vi "Get Core Configuration.vi"(8 "error in":errorcluster, 11 "custom device":T1 format="%.0x") -> (0 "error out":errorcluster, 2 "configuration string":string, 3 "custom device out":T1 format="%.0x")   [LabVIEW 2020, in "Ballard ARINC 429 Hardware Configuration.lvlib"]
uses:
  Ballard ARINC 429 Hardware Configuration.lvlib
  <vilib>/NI VeriStand/Custom Device API/Custom Device Item Ref.ctl
  Constants.vi
  Scripting/Ballard/Ballard ARINC 429 Scripting.lvlib
  <vilib>/NI VeriStand/Custom Device API/Custom Device API.lvlib
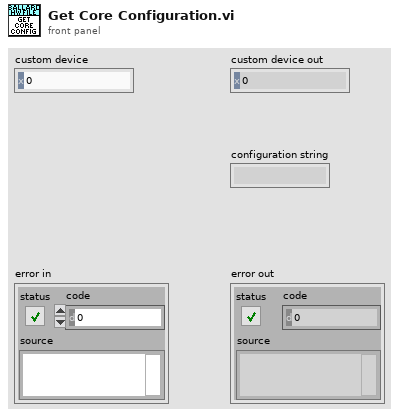
[diagram p1: front panel]
types:
  T1 = typedef "Custom Device API.lvlib/Custom Device Item Ref.ctl" = u64
  T2 = typedef "Device Parameters.ctl" = cluster{"initialization method":T3, "card number":i32, "PXI slot number":i32, "core number":i32}
  T3 = typedef "Initialization Method.ctl" = enum16{"PXI Slot Number", "Card Number"}
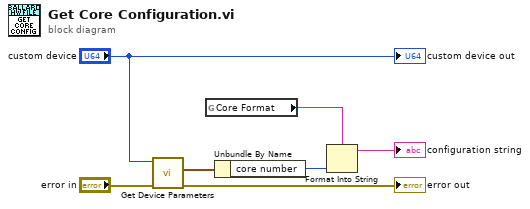
[diagram p0: block diagram]
diagram:
  n1 = call "Get Device Parameters.vi"("error in"="error in", "Ballard ARINC 429 custom device in"="custom device") -> ("error out"=→"error out":errorcluster, "device parameters"=w4:T2)  [unwired: 7 in, 1 out]
  n2 = global read "Constants.vi" "Core Format"() -> (w3:string)
  n3 = Unbundle By Name(w4) -> ("core number"=w2:i32)
  n4 = Format Into String(format string=w3, w2) -> (resulting string=→"configuration string":string)  [unwired: 2 in, 1 out]
  "custom device out" <- "custom device"
